vi "A test results.vi"(0 "Fitted Circle (Find Circular Edge 1)":T1 {"Average SNR (dB)" format="%.2f"; "Average Strength" format="%.2f"; "Roundness (Real-World)" format="%.2f"; "Radius (Real-World)" format="%.2f"; "Center (Real-World)"."Y" format="%.2f"; "Center (Real-World)"."X" format="%.2f"; "Radius (Pixels)" format="%.2f"; "Center (Pixels)"."Y" format="%.2f"; "Center (Pixels)"."X" format="%.2f"}, 2 "Tbl引用句柄":refnum<vi>, 3 "error in (no error)":errorcluster caption="错误输入（无错误）") -> (10 "error out":errorcluster caption="错误输出")   [LabVIEW 2017]
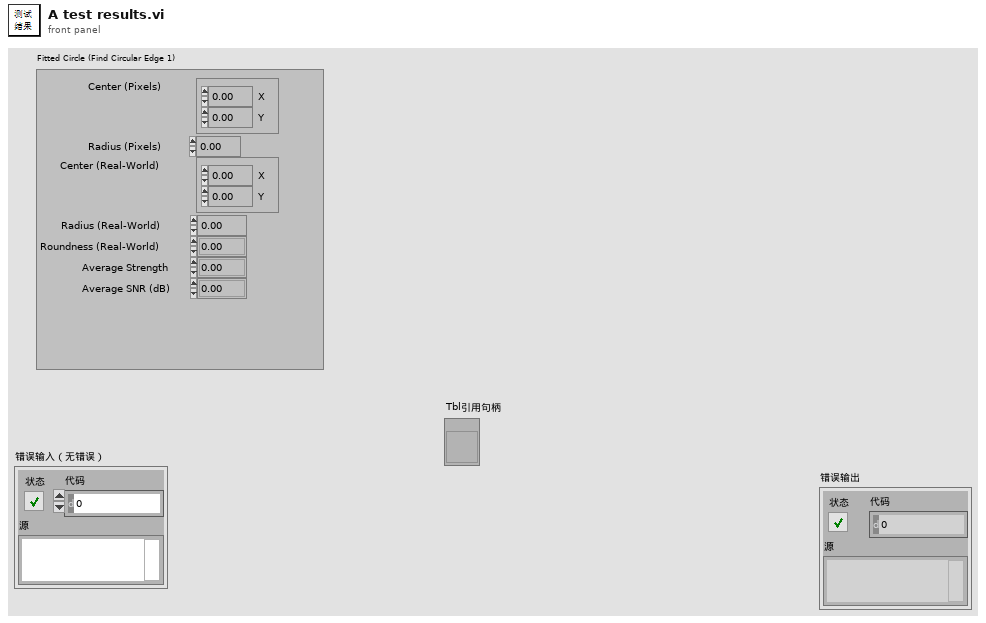
[diagram p1: front panel]
types:
  T1 = cluster{"Center (Pixels)":cluster{"X":sgl, "Y":sgl}, "Radius (Pixels)":dbl, "Center (Real-World)":cluster{"X":sgl, "Y":sgl}, "Radius (Real-World)":dbl, "Roundness (Real-World)":dbl, "Average Strength":dbl, "Average SNR (dB)":dbl}
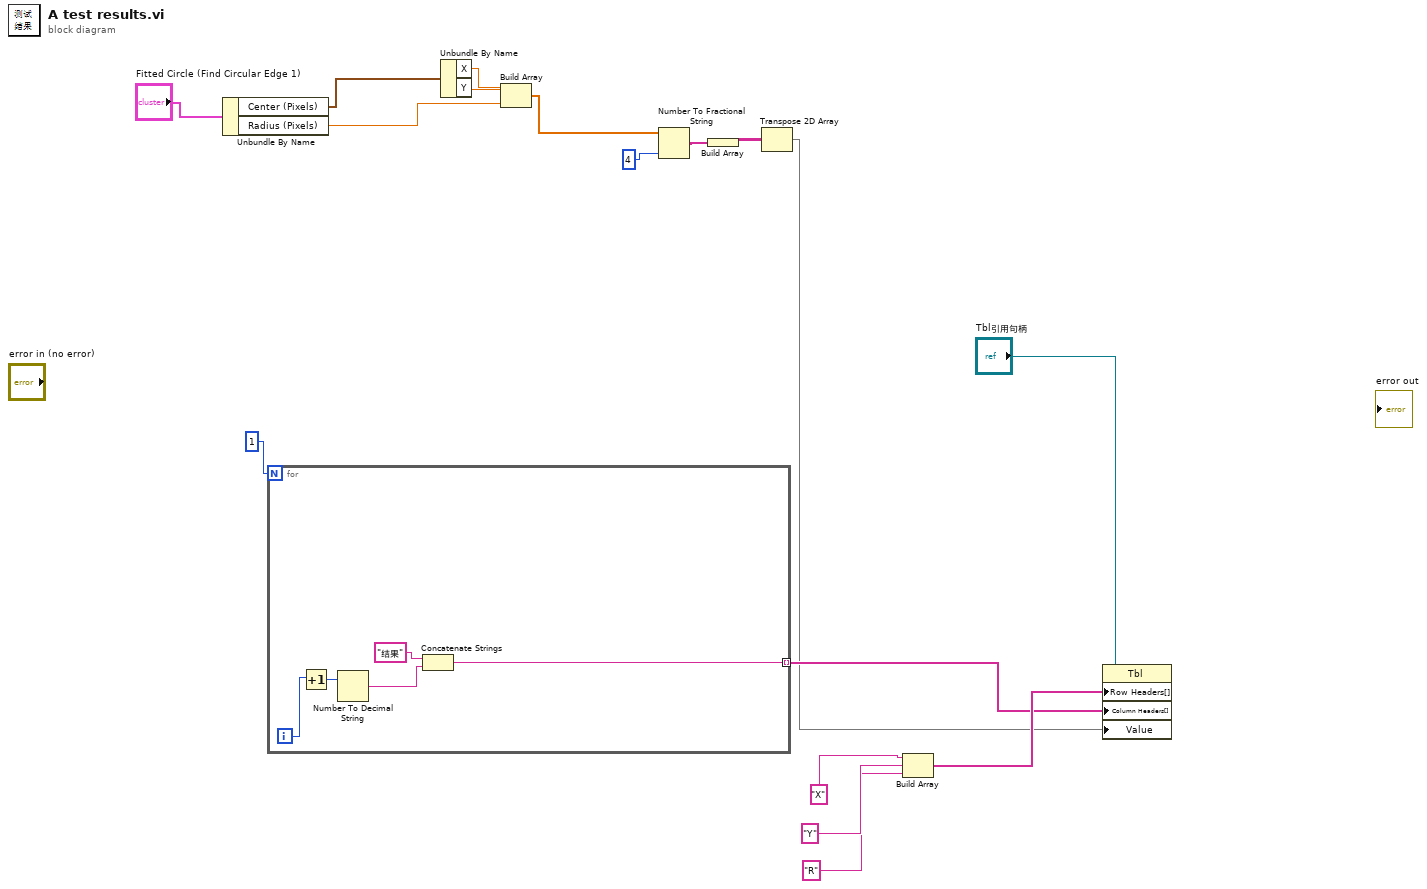
[diagram p0: block diagram]
diagram:
  n1 = Unbundle By Name("Fitted Circle (Find Circular Edge 1)") -> ("Center (Pixels)"=w9:cluster{"X":sgl, "Y":sgl}, "Radius (Pixels)"=w6:dbl)
  n2 = for {
    N: 1 -> [_]
    tunnel: [w20] -> w13 mode=indexing
    i -> [w19]
    n3 = Increment(x=w19) -> (x+1=w18:i32)
    n4 = Number To Decimal String(number=w18) -> (decimal integer string=w21:string)  [unwired: 1 in]
    n5 = Concatenate Strings("结果", w21) -> (w20:string)
  }
  n6 = Unbundle By Name(w9) -> ("X"=w8:sgl, "Y"=w7:sgl)
  n7 = Build Array(w8, w7, w6) -> (w4:dbl[])
  n8 = Number To Fractional String(number=w4, precision (6)=i16 4 ("精度(6)")) -> (F-format string=w3:string[])  [unwired: 2 in]
  n9 = Build Array(w3) -> (w2:string[][])
  n10 = Transpose 2D Array(2D array=w2) -> (transposed array=w1:string[][])
  n11 = Build Array("X", "Y" ("元素"), "R" ("元素")) -> (w15:string[])
  n12 = property class="Tbl"(reference="Tbl引用句柄", "Row Headers[]"=w15, "Column Headers[]"=w13, "Value"=w1) -> ()  [unwired: 1 in, 2 out]
